vi "configure.vi"(8 "error in (no error)":errorcluster, 11 "DAQ  in":refnum<class "DAQ .lvclass">) -> (0 "error out":errorcluster, 3 "DAQ  out":refnum<class "DAQ .lvclass">)   [LabVIEW 2026, in "Hardware.lvlib" / "DAQ .lvclass"]
uses:
  DAQ .lvclass
  C:/Users/E2013170/Documents/GitHub/Measurement-Utility-Reference/components/MAL-Framework/user.lib/Common Components/Hardware/Hardware.lvclass
  config/DAQ Configuration.lvclass
  MAL-Framework/user.lib/Common Components/Hardware/Hardware.lvclass/Hardware.ctl
  config/DAQ Configuration.lvclass/DAQ Configuration.ctl
  DAQ .lvclass/DAQ .ctl
  <vilib>/DAQmx/create/channels.llb/DAQmx Create Channel (AI-Current-Basic).vi
  <vilib>/DAQmx/create/channels.llb/DAQmx Create Channel (AI-Voltage-Basic).vi
  <vilib>/DAQmx/create/channels.llb/DAQmx Create Channel (AI-Temperature-Thermocouple).vi
  <vilib>/DAQmx/configure/timing.llb/DAQmx Timing (Sample Clock).vi
  MAL-Framework/user.lib/Common Components/Hardware/Hardware.lvclass
  MAL-Framework/user.lib/Common Components/Hardware/HW Config/HW Configuration.lvclass
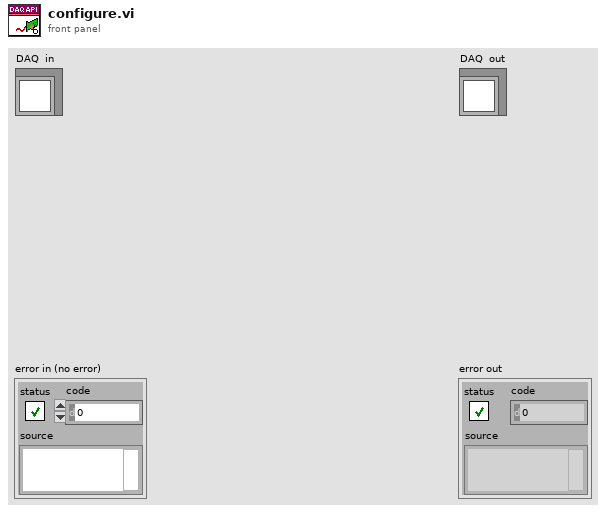
[diagram p1: front panel]
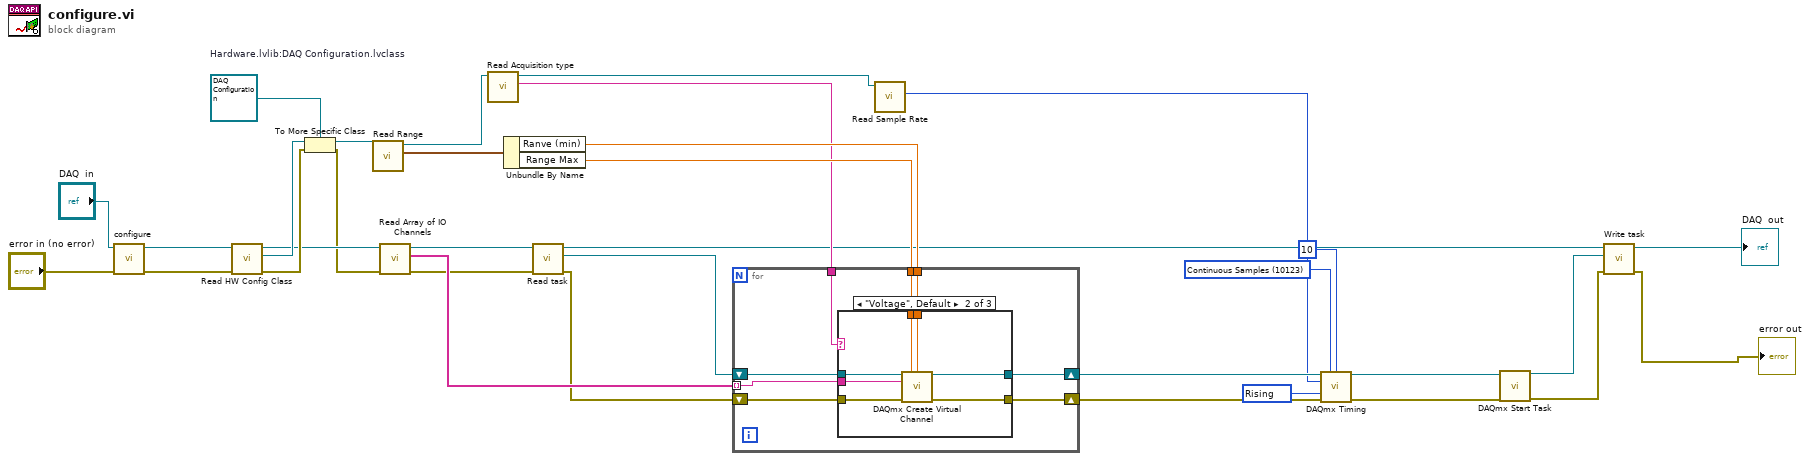
[diagram p0: block diagram]
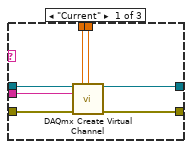
[diagram p2: hidden frame]
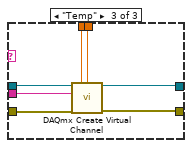
[diagram p3: hidden frame]
diagram:
  w18 = refnum<class "DAQ Configuration.lvclass"> refnum  # Hardware.lvlib:DAQ Configuration.lvclass
  w22 = 10123 items=["Finite Samples"=10178, "Continuous Samples"=10123, "Hardware Timed Single Point"=12522] ("sample mode")
  w23 = 10280 items=["Rising"=10280, "Falling"=10171] ("active edge")
  n1 = call-parent "configure.vi"("error in (no error)"="error in (no error)", "Hardware in"="DAQ  in") -> ("error out"=w31:errorcluster, "Hardware out"=w32:refnum<class "DAQ .lvclass">)  [unwired: 8 in]
  n2 = call "Read HW Config Class.vi"("error in (no error)"=w31, "Hardware in"=w32) -> ("error out"=w17:errorcluster, "Hardware.lvlib:HW Configuration.lvclass"=w19:refnum<class "HW Configuration.lvclass">, "Hardware out"=w12:refnum<class "DAQ .lvclass">)  [unwired: 7 in]
  n3 = To More Specific Class(target class=w18, reference=w19, error in=w17) -> (specific class reference=w16:refnum<class "DAQ Configuration.lvclass">, error out=w11:errorcluster)
  n4 = call "Read Range.vi"("DAQ Configuration in"=w16) -> ("Range"=w15:cluster{"Ranve (min)":dbl, "Range Max":dbl}, "DAQ Configuration out"=w9:refnum<class "DAQ Configuration.lvclass">)  [unwired: 8 in, 1 out]
  n5 = call "Read Array of IO Channels.vi"("error in (no error)"=w11, "Hardware in"=w12) -> ("error out"=w6:errorcluster, "Array of IO Channels"=w10:string[], "Hardware out"=w7:refnum<class "DAQ .lvclass">)  [unwired: 7 in]
  n6 = call "Read Acquisition type.vi"("DAQ Configuration in"=w9) -> ("Acquisition type"=w8:string, "DAQ Configuration out"=w2:refnum<class "DAQ Configuration.lvclass">)  [unwired: 8 in, 1 out]
  n7 = Unbundle By Name(w15) -> ("Ranve (min)"=w13:dbl, "Range Max"=w14:dbl)
  n8 = call "Read task.vi"("error in (no error)"=w6, "DAQ  in"=w7) -> ("error out"=w5:errorcluster, "task"=w4:refnum<k21>, "DAQ  out"=w3:refnum<class "DAQ .lvclass">)  [unwired: 7 in]
  n9 = for {
    tunnel: w14 -> [w38]
    tunnel: w13 -> [w37]
    shift-right: [w41] -> w28
    shift-left: w4 -> [w42]
    shift-right: [w39] -> w26
    shift-left: w5 -> [w40]
    tunnel: w10 -> [w36] mode=indexing
    tunnel: w8 -> [w35]
    n10 = case shown="\"Voltage\", Default" w35 {
      tunnel: w42 -> [w49 w56 w61]
      tunnel: [w46 w55 w57] -> w41
      tunnel: w40 -> [w48 w54 w59]
      tunnel: [w47 w53 w58] -> w39
      tunnel: w38 -> [w45 w52 w63]
      tunnel: w37 -> [w44 w51 w62]
      tunnel: w36 -> [w43 w50 w60]
      frame "Current" {
        n11 = call-poly <vilib>:"DAQmx Create Virtual Channel.vi"("task in"=w49, "maximum value"=w45, "minimum value"=w44, "physical channels"=w43, "error in"=w48) -> ("task out"=w46:refnum<k21>, "error out"=w47:errorcluster)  [unwired: 9 in]
      }
      frame "Voltage", Default {
        n12 = call-poly <vilib>:"DAQmx Create Virtual Channel.vi"("task in"=w56, "maximum value"=w52, "minimum value"=w51, "physical channels"=w50, "error in"=w54) -> ("task out"=w55:refnum<k21>, "error out"=w53:errorcluster)  [unwired: 9 in]
      }
      frame "Temp" {
        n13 = call-poly <vilib>:"DAQmx Create Virtual Channel.vi"("task in"=w61, "maximum value"=w63, "minimum value"=w62, "physical channels"=w60, "error in"=w59) -> ("task out"=w57:refnum<k21>, "error out"=w58:errorcluster)  [unwired: 9 in]
      }
    }
  }
  n14 = call "Read Sample Rate.vi"("DAQ Configuration in"=w2) -> ("Sample Rate"=w1:i32)  [unwired: 8 in, 2 out]
  n15 = call-poly <vilib>:"DAQmx Timing.vi"("task/channels in"=w28, "sample mode"=w22, "samples per channel"=10, "rate"=w1, "active edge"=w23, "error in"=w26) -> ("task out"=w27:refnum<k21>, "error out"=w25:errorcluster)  [unwired: 8 in]
  n16 = call <vilib>:"DAQmx Start Task.vi"("task/channels in"=w27, "error in"=w25) -> ("task out"=w20:refnum<k21>, "error out"=w24:errorcluster)  [unwired: 12 in]
  n17 = call "Write task.vi"("error in (no error)"=w24, "task"=w20, "DAQ  in"=w3) -> ("error out"=→"error out":errorcluster, "DAQ  out"=→"DAQ  out":refnum<class "DAQ .lvclass">)  [unwired: 7 in]
